vi "tempDAQ.vi"() -> ()   [LabVIEW 2015]
uses:
  globals.vi
  output_byte.vi
panel:
  out "Numeric":dbl
  out "Motors Out":bool[](array[boolean])
  in  "Outputs (digital)":tag
  out "Switches In":bool[](array[boolean])
  in  "Switches (digital)":tag
  out "shoulder angle":dbl
  out "Shoulder Angle":dbl(knob) scale=0.0..180.0
  out "Sh Max voltage":dbl
  out "Sh Min voltage":dbl
  out "Elbow Angle":dbl(knob) scale=0.0..180.0
  out "elbow angle":dbl
  out "El Max voltage":dbl
  out "El Min voltage":dbl
  in  "stop":bool
  in  "Potentiometers (ADC)":tag
  # "use Dev1/ai0:7"
  # "use Dev1/port1"
  # "use Dev1/port0"
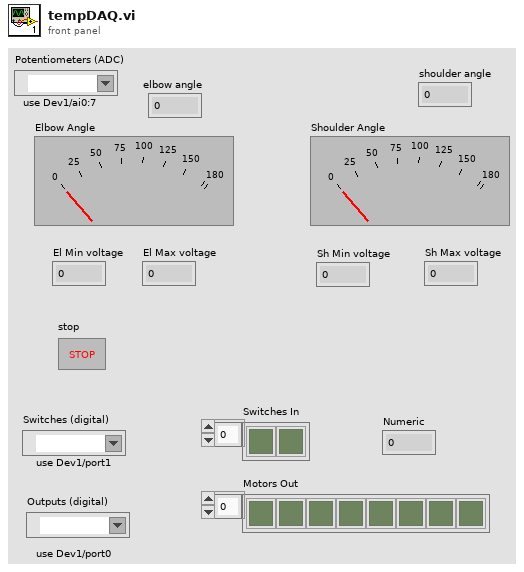
[diagram p1: front panel]
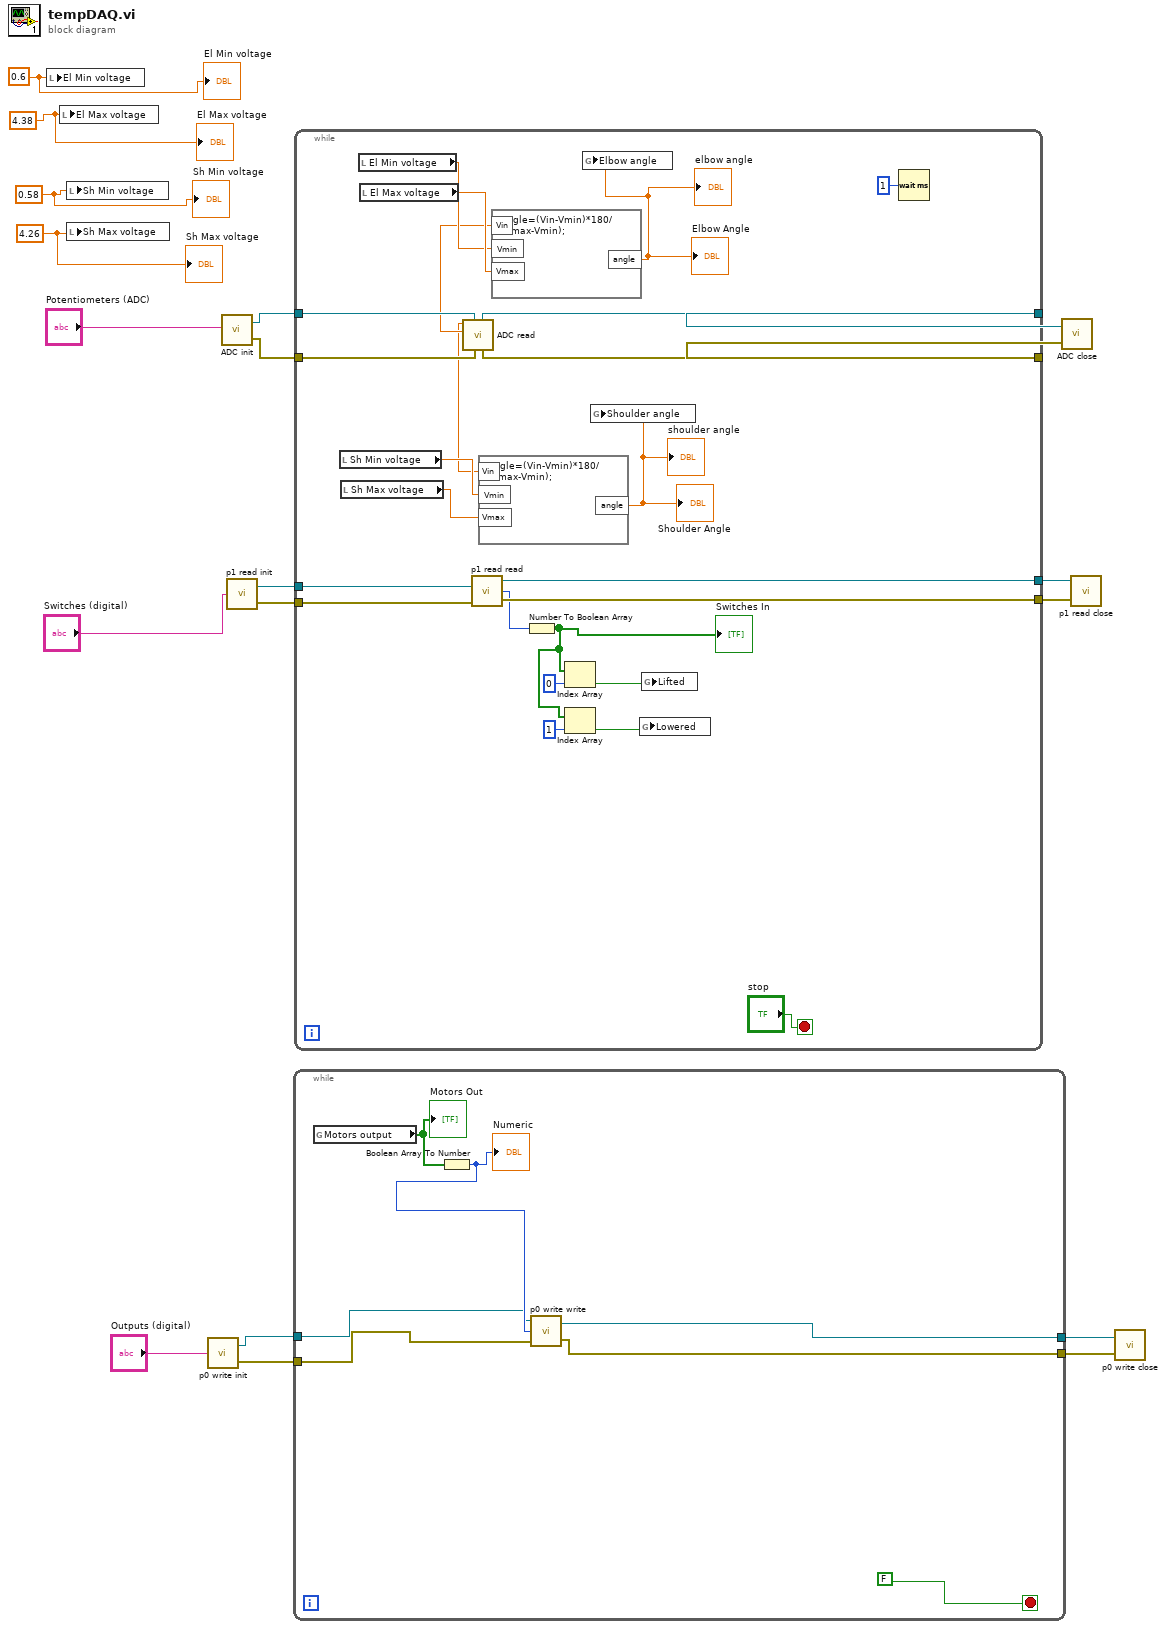
[diagram p0: block diagram]
diagram:
  w11 = 4.26
  w12 = 0.58
  w14 = 4.38
  w13 = 0.6
  n1 = local write "El Min voltage"(w13) -> ()
  n2 = local write "El Max voltage"(w14) -> ()
  n3 = local write "Sh Min voltage"(w12) -> ()
  n4 = local write "Sh Max voltage"(w11) -> ()
  n5 = call "p0 write init.vi"("Port"="Outputs (digital)") -> ("task out"=w4:refnum<k21>, "error out"=w3:errorcluster)
  n6 = call "ADC init.vi"("Physical Channel"="Potentiometers (ADC)") -> ("task out"=w18:refnum<k21>, "error out"=w17:errorcluster)
  n7 = call "p1 read init.vi"("Port"="Switches (digital)") -> ("task out"=w7:refnum<k21>, "error out"=w9:errorcluster)
  n8 = while {
    tunnel: w4 -> [w23]
    tunnel: w3 -> [w22]
    tunnel: [w21] -> w2
    tunnel: [w20] -> w1
    stop <- FALSE stop-if-true
    n9 = global read "output_byte.vi" "Motors output"() -> (w26:bool[])
    "Motors Out" <- w26
    n10 = Boolean Array To Number(Boolean array=w26) -> (number=w24:u32)
    "Numeric" <- w24
    n11 = call "p0 write write.vi"("error in"=w22, "Data to Write"=w24, "task/channels in"=w23) -> ("error out"=w21:errorcluster, "task out"=w20:refnum<k21>)
  }
  n12 = while {
    tunnel: w18 -> [w50]
    tunnel: w17 -> [w49]
    tunnel: [w48] -> w16
    tunnel: [w47] -> w15
    tunnel: [w37] -> w10
    tunnel: w9 -> [w36]
    tunnel: w7 -> [w35]
    tunnel: [w34] -> w6
    stop <- "stop" stop-if-true
    n13 = local read "Sh Min voltage"() -> (w41:dbl)
    n14 = local read "Sh Max voltage"() -> (w40:dbl)
    n15 = local read "El Min voltage"() -> (w45:dbl)
    n16 = local read "El Max voltage"() -> (w46:dbl)
    n17 = call "ADC read.vi"("error in"=w49, "task/channels in"=w50) -> ("error out"=w47:errorcluster, "task out"=w48:refnum<k21>, "adc1"=w42:dbl, "adc0"=w39:dbl)  [unwired: 6 out]
    n18 = call "p1 read read.vi"("task in"=w35, "error in"=w36) -> ("task out"=w34:refnum<k21>, "Data Read"=w33:u32, "error out"=w37:errorcluster)
    n19 = formula code="angle=(Vin-Vmin)*180/(Vmax-Vmin);"("Vin"=w39, "Vmin"=w41, "Vmax"=w40) -> ("angle"=w38:dbl)
    "Shoulder Angle" <- w38
    "shoulder angle" <- w38
    n20 = formula code="angle=(Vin-Vmin)*180/(Vmax-Vmin);"("Vin"=w42, "Vmin"=w45, "Vmax"=w46) -> ("angle"=w44:dbl)
    "elbow angle" <- w44
    "Elbow Angle" <- w44
    n21 = Number To Boolean Array(number=w33) -> (Boolean array=w30:bool[])
    "Switches In" <- w30
    n22 = Index Array(array=w30, index=0) -> (element=w29:bool)
    n23 = Index Array(array=w30, index=1) -> (element=w28:bool)
    n24 = global write "globals.vi" "Elbow angle"(w44) -> ()
    n25 = global write "globals.vi" "Shoulder angle"(w38) -> ()
    n26 = global write "globals.vi" "Lowered"(w28) -> ()
    n27 = global write "globals.vi" "Lifted"(w29) -> ()
    n28 = Wait (ms)(milliseconds to wait=u32 1) -> ()  [unwired: 1 out]
  }
  n29 = call "ADC close.vi"("error in"=w15, "task/channels in"=w16) -> ()
  n30 = call "p1 read close.vi"("error in"=w10, "task in"=w6) -> ()
  n31 = call "p0 write close.vi"("error in"=w2, "task/channels in"=w1) -> ()
  "El Min voltage" <- w13
  "El Max voltage" <- w14
  "Sh Min voltage" <- w12
  "Sh Max voltage" <- w11
